vi "Write Menue 2.vi"(8 "error in (no error)":errorcluster, 10 "Menue 2":refnum<user-event>, 11 "MenueItem in":refnum<class "MenueItem.lvclass">) -> (0 "error out":errorcluster, 3 "MenueItem out":refnum<class "MenueItem.lvclass">)   [LabVIEW 2016, in "MenueItem.lvclass"]
uses:
  MenueItem.lvclass
  MenueItem.lvclass/MenueItem.ctl
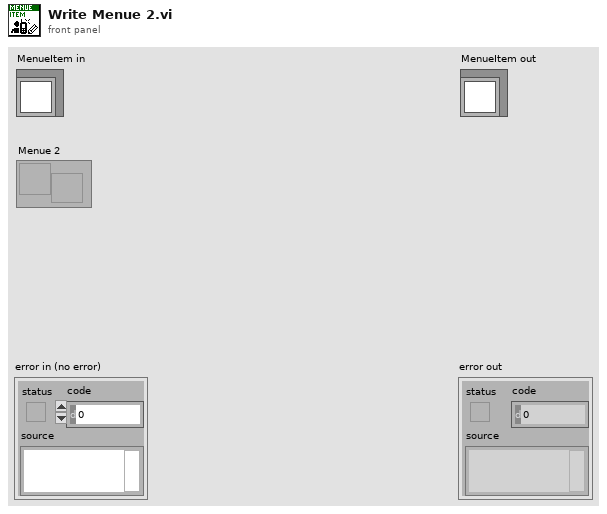
[diagram p1: front panel]
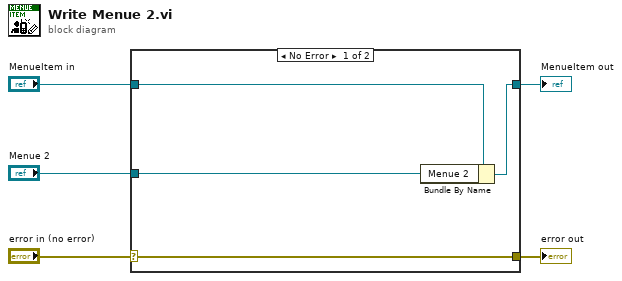
[diagram p0: block diagram]
diagram:
  n1 = case shown="No Error" "error in (no error)" {
    selector: "error in (no error)" -> [w9 w10]
    tunnel: [w9 w10] -> w4
    tunnel: [w7 w11] -> w2
    tunnel: "MenueItem in" -> [w8 w11]
    tunnel: "Menue 2" -> [w6 _]
    frame No Error {
      n2 = Bundle By Name(cluster=w8, "Menue 2"=w6) -> (w7:refnum<class "MenueItem.lvclass">)
    }
    frame Error {
    }
  }
  "error out" <- w4
  "MenueItem out" <- w2
